vi "Set Main Ctl and VI Reference.vi"(8 "error in (no error)":errorcluster, 10 "Main Ctl and VI Refenerence":T1, 11 "Actor in":refnum<class "Actor.lvclass">) -> (0 "error out":errorcluster, 3 "Actor out":refnum<class "Actor.lvclass">)   [LabVIEW 2015, in "Actor.lvclass"]
uses:
  Actor.lvclass
  Type Definition/Main Ctl and VI Refenerce.ctl
  Actor.lvclass/Actor.ctl
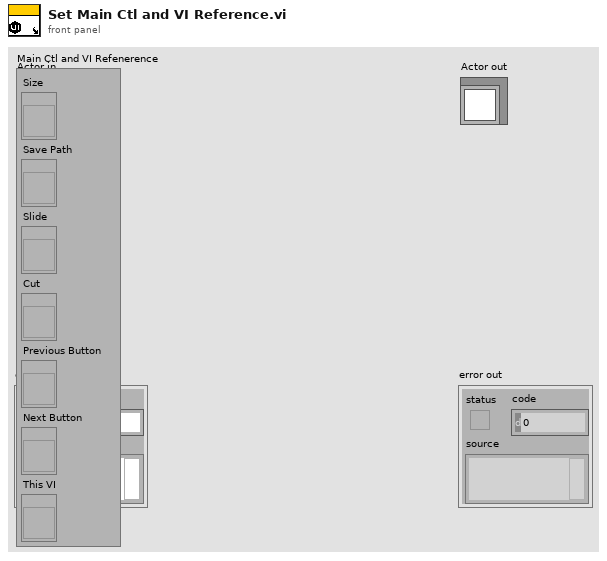
[diagram p1: front panel]
types:
  T1 = typedef "Actor.lvclass/Main Ctl and VI Refenerce.ctl" = cluster{"Size":refnum<vi>, "Save Path":refnum<vi>, "Slide":refnum<vi>, "Cut":refnum<vi>, "Previous Button":refnum<vi>, "Next Button":refnum<vi>, "This VI":refnum<vi>}
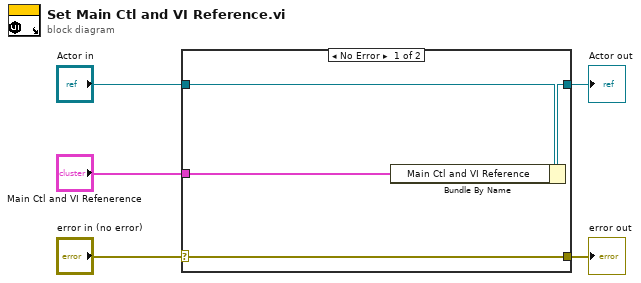
[diagram p0: block diagram]
diagram:
  n1 = case shown="No Error" "error in (no error)" {
    selector: "error in (no error)" -> [w9 w10]
    tunnel: [w9 w10] -> w4
    tunnel: [w7 w11] -> w2
    tunnel: "Actor in" -> [w8 w11]
    tunnel: "Main Ctl and VI Refenerence" -> [w6 _]
    frame No Error {
      n2 = Bundle By Name(cluster=w8, "Main Ctl and VI Reference"=w6) -> (w7:refnum<class "Actor.lvclass">)
    }
    frame Error {
    }
  }
  "error out" <- w4
  "Actor out" <- w2
